vi "AVS_SetSensitivityMode.vi"(0 "a_hDevice":i32, 7 "a_SensitivityMode":u32) -> (4 "Output Value":i32)   [LabVIEW 2016]
uses:
  libavs.so
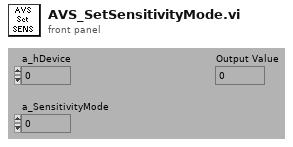
[diagram p1: front panel]
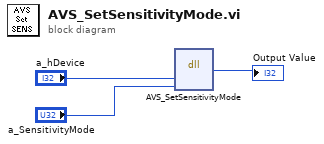
[diagram p0: block diagram]
diagram:
  n1 = dll-call lib="home/harini/tcs/ts_sedspectrometer/ss_sedspectrometer/VIs/libavs.so" fn="AVS_SetSensitivityMode"("a_hDevice"="a_hDevice", "a_SensitivityMode"="a_SensitivityMode") -> ("return type"=→"Output Value":i32)  [unwired: 5 in, 2 out]
